vi "CheckNTDataEnd.vi"(10 "GetData":bool, 11 "ValToCheck":dbl) -> ()   [LabVIEW 2018]
uses:
  <vilib>/Rock Robotics/Network Tables/NT Write Boolean.vi
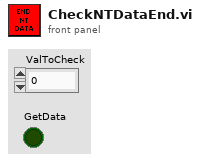
[diagram p1: front panel]
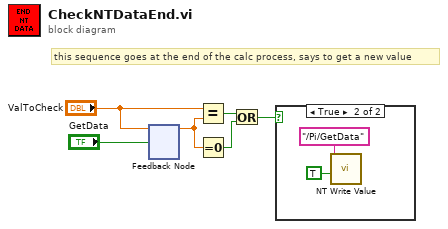
[diagram p0: block diagram]
diagram:
  # "this sequence goes at the end of the calc process, says to get a new value"
  n1 = feedback #1() -> (w6:dbl)  [unwired: 1 in]
  n2 = feedback-in #1("ValToCheck", "GetData") -> ()
  n3 = Equal?(x="ValToCheck", y=w6) -> (x = y?=w5:bool)
  n4 = Equal To 0?(x=w6) -> (x = 0?=w4:bool)
  n5 = Or(x=w5, y=w4) -> (x .or. y?=w3:bool)
  n6 = case shown="True" w3 {
    frame False {
    }
    frame True {
      n7 = call-poly <vilib>:"NT Write Value.vi"("Boolean"=TRUE, "Name"="/Pi/GetData" ("Client Name")) -> ()  [unwired: 9 in, 1 out]
    }
  }
